vi "Get log paths.vi"(11 "Chamber ID":T1={"Chamber name"="Analysis", "Trip pressure"=5e-07}) -> (3 "paths":string)   [LabVIEW 2019, in "PGC2D.lvlib"]
uses:
  PGC2D.lvlib
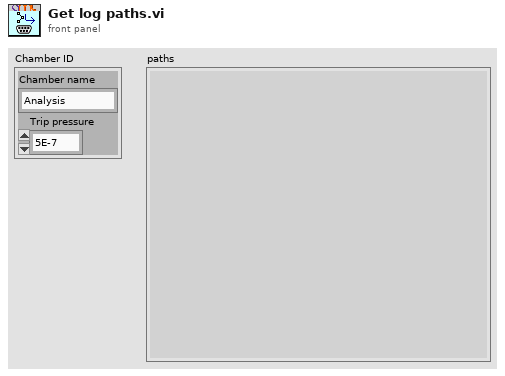
[diagram p1: front panel]
types:
  T1 = cluster{"Chamber name":string, "Trip pressure":dbl}
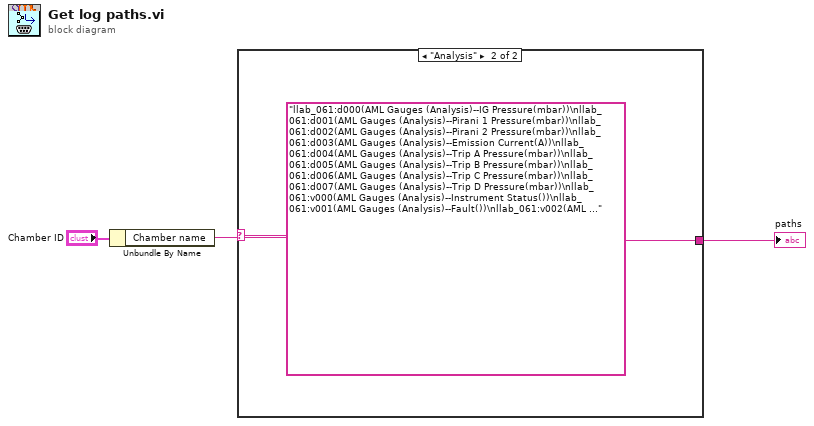
[diagram p0: block diagram]
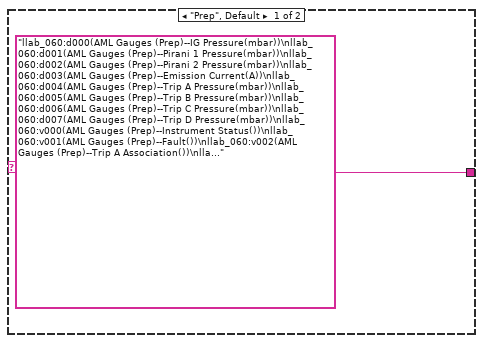
[diagram p2: hidden frame]
diagram:
  n1 = Unbundle By Name("Chamber ID") -> ("Chamber name"=w1:string)
  n2 = case shown="\"Analysis\"" w1 {
    tunnel: ["llab_060:d000(AML Gauges (Prep)--IG Pressure(mbar))\nllab_060:d001(AML Gauges (Prep)--Pirani 1 Pressure(mbar))\nllab_060:d002(AML Gauges (Prep)--Pirani 2 Pressure(mbar))\nllab_060:d003(AML Gauges (Prep)--Emission Current(A))\nllab_060:d004(AML Gauges (Prep)--Trip A Pressure(mbar))\nllab_060:d005(AML Gauges (Prep)--Trip B Pressure(mbar))\nllab_060:d006(AML Gauges (Prep)--Trip C Pressure(mbar))\nllab_060:d007(AML Gauges (Prep)--Trip D Pressure(mbar))\nllab_060:v000(AML Gauges (Prep)--Instrument Status())\nllab_060:v001(AML Gauges (Prep)--Fault())\nllab_060:v002(AML Gauges (Prep)--Trip A Association())\nllab_060:v003(AML Gauges (Prep)--Trip B Association())\nllab_060:v004(AML Gauges (Prep)--Trip C Association())\nllab_060:v005(AML Gauges (Prep)--Trip D Association())\nllab_060:v006(AML Gauges (Prep)--Relay A())\nllab_060:v007(AML Gauges (Prep)--Relay B())\nllab_060:v008(AML Gauges (Prep)--Relay C())\nllab_060:v009(AML Gauges (Prep)--Relay D())" "llab_061:d000(AML Gauges (Analysis)--IG Pressure(mbar))\nllab_061:d001(AML Gauges (Analysis)--Pirani 1 Pressure(mbar))\nllab_061:d002(AML Gauges (Analysis)--Pirani 2 Pressure(mbar))\nllab_061:d003(AML Gauges (Analysis)--Emission Current(A))\nllab_061:d004(AML Gauges (Analysis)--Trip A Pressure(mbar))\nllab_061:d005(AML Gauges (Analysis)--Trip B Pressure(mbar))\nllab_061:d006(AML Gauges (Analysis)--Trip C Pressure(mbar))\nllab_061:d007(AML Gauges (Analysis)--Trip D Pressure(mbar))\nllab_061:v000(AML Gauges (Analysis)--Instrument Status())\nllab_061:v001(AML Gauges (Analysis)--Fault())\nllab_061:v002(AML Gauges (Analysis)--Trip A Association())\nllab_061:v003(AML Gauges (Analysis)--Trip B Association())\nllab_061:v004(AML Gauges (Analysis)--Trip C Association())\nllab_061:v005(AML Gauges (Analysis)--Trip D Association())\nllab_061:v006(AML Gauges (Analysis)--Relay A())\nllab_061:v007(AML Gauges (Analysis)--Relay B())\nllab_061:v008(AML Gauges (Analysis)--Relay C())\nllab_061:v009(AML Gauges (Analysis)--Relay D())"] -> w2
    frame "Prep", Default {
    }
    frame "Analysis" {
    }
  }
  "paths" <- w2
